vi "move_4.vi"(6 "Array 3":i32[](array[numeric]), 7 "Array 6":i32[](array[numeric]), 9 "Array in":i32[](array[numeric]), 10 "Enum 4":T1(ring), 11 "Enum in":enum16{"move4", "move4_1", "move4_2"}(ring)) -> (1 "Array out":i32[](array[numeric]), 2 "Enum 3":T2(ring), 3 "Enum out":enum16{"move4", "move4_1", "move4_2"}(ring), 4 "Array 4":i32[](array[numeric]), 5 "Array 5":i32[](array[numeric]))   [LabVIEW 2016]
uses:
  <vilib>/NXT/Block Support/NXT_OutputPort.ctl
  <vilib>/NXT/NXTIO Xnodes/NXTIONodeSubVIs/NXTStopMotors.vi
  <vilib>/NXT/NXTIO Xnodes/NXTIONodeSubVIs/NXTMotorRunDistance.vi
  <vilib>/NXT/NXTIO Xnodes/NXTIONodeSubVIs/LEGOMotorStatus.vi
  <vilib>/NXT/NXTIO Xnodes/NXTIONodeSubVIs/NXTMoveMotors.vi
  <vilib>/NXT/NXTIO Xnodes/NXTIONodeSubVIs/LEGOResetMotors.vi
  <vilib>/NXT/Subs/LVHSConnector.ctl
  <vilib>/NXT/NXTIO Xnodes/AddressXNode/NXTIOAddress.xnode
  <vilib>/NXT/NXTIO Xnodes/NXTIOXNode/NXTIO.xnode
  <vilib>/NXT/LegoClasses/BrickReference/BrickReference.lvclass
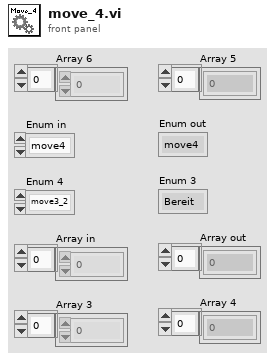
[diagram p1: front panel]
types:
  T1 = enum16{"move3_2", "move3_3", "move3_4", "move3_5"}
  T2 = enum16{"Bereit", "Move 1", "Reference_pos", "Wait", "row1_check", "row2_check", "row3_check", "return", "move2", "move3", "move4", "move5", "end"}
  T3 = enum16{"forward", "right", "mark", "pause", "up", "return", "end"}
  T4 = typedef "NXT_OutputPort.ctl" = u8
  T5 = cluster{"Output Port":T4, "Output Port 2":T4, "Output Port 3":T4}
  T6 = enum16{"forward", "mark", "pause", "up", "return", "end"}
  T7 = typedef "LVHSConnector.ctl" = refnum<class "BrickReference.lvclass">
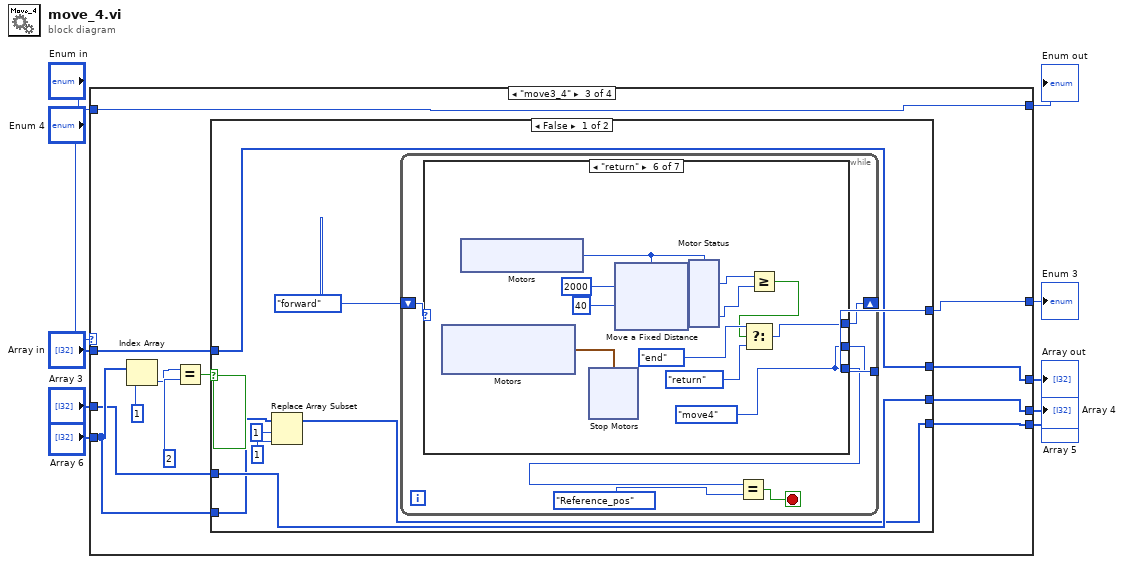
[diagram p0: block diagram]
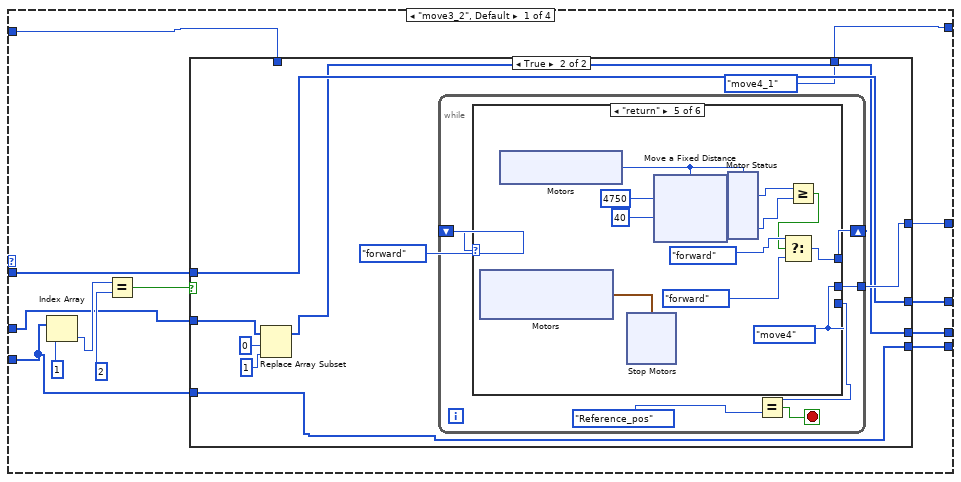
[diagram p2: hidden frame]
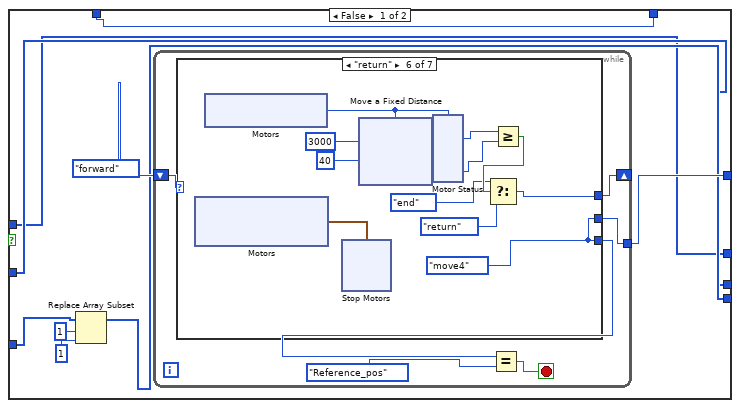
[diagram p3: hidden frame]
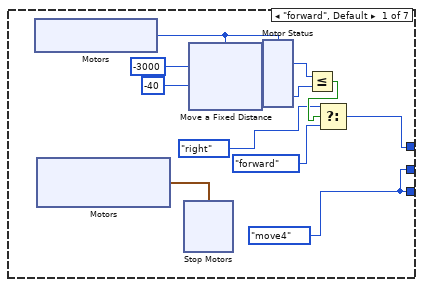
[diagram p4: hidden frame]
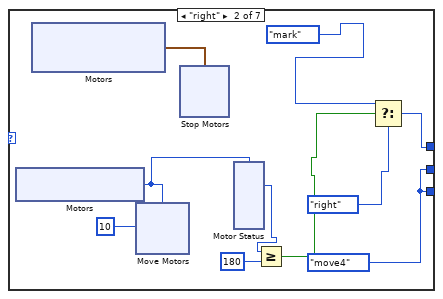
[diagram p5: hidden frame]
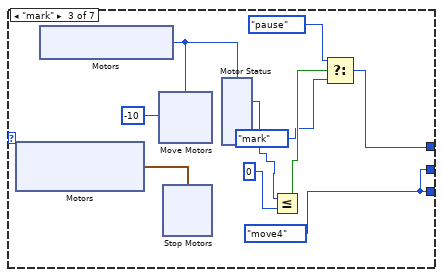
[diagram p6: hidden frame]
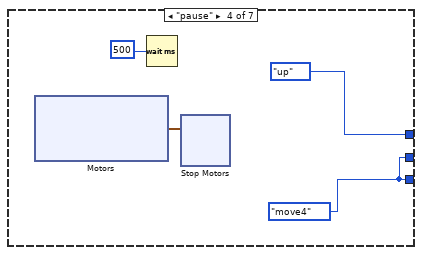
[diagram p7: hidden frame]
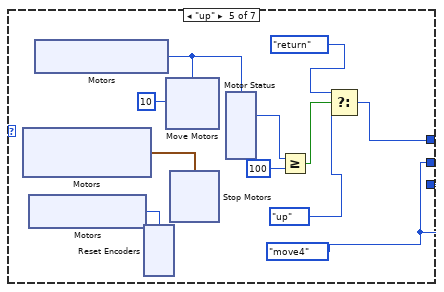
[diagram p8: hidden frame]
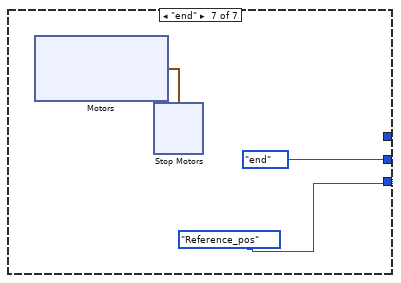
[diagram p9: hidden frame]
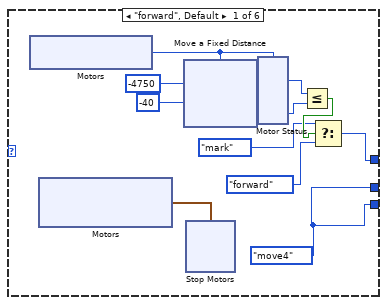
[diagram p10: hidden frame]
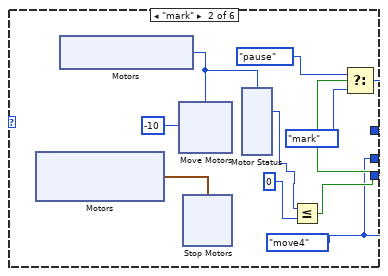
[diagram p11: hidden frame]
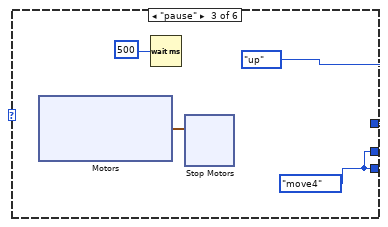
[diagram p12: hidden frame]
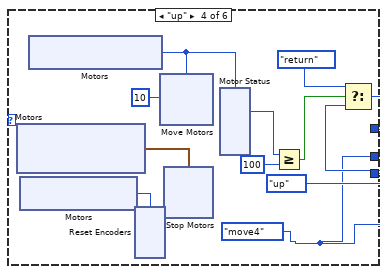
[diagram p13: hidden frame]
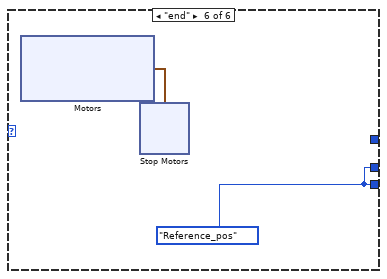
[diagram p14: hidden frame]
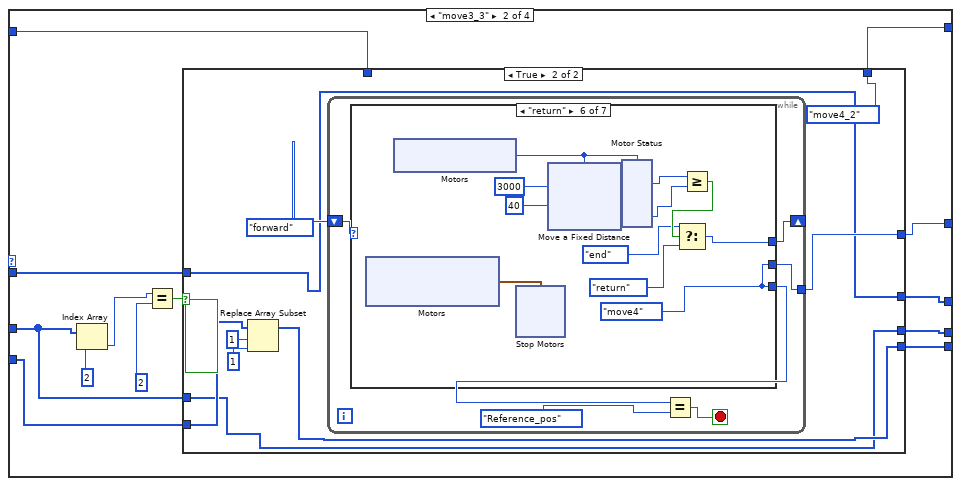
[diagram p15: hidden frame]
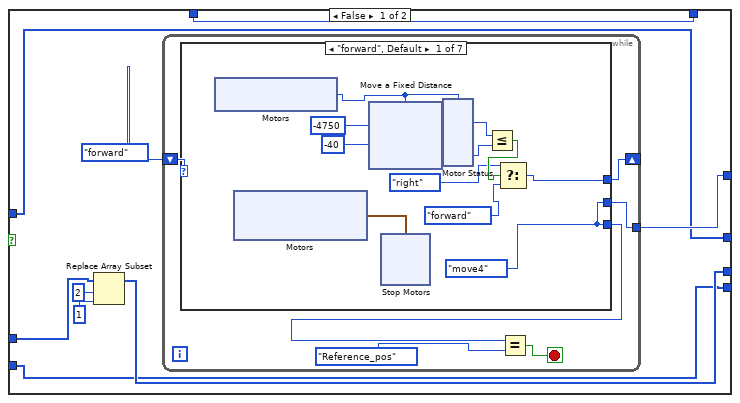
[diagram p16: hidden frame]
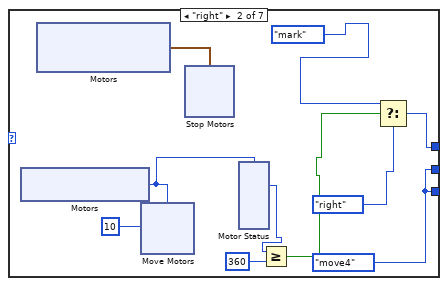
[diagram p17: hidden frame]
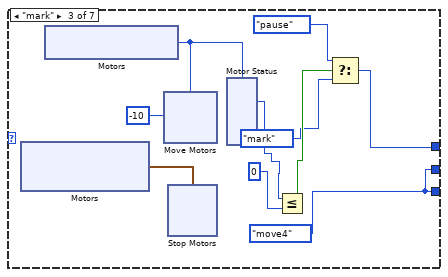
[diagram p18: hidden frame]
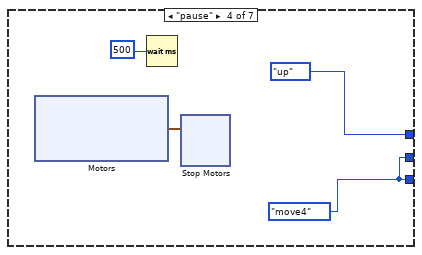
[diagram p19: hidden frame]
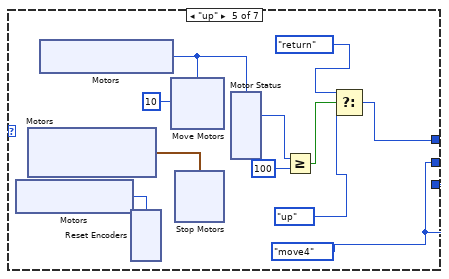
[diagram p20: hidden frame]
diagram:
  n1 = case shown="\"move3_4\"" "Enum 4" {
    tunnel: [w22 w417 w844 w1236] -> w2
    tunnel: [w12 w408 w835 w1227] -> w3
    tunnel: "Enum in" -> [w11 w407 w835 w1227]
    tunnel: "Array 6" -> [w18 w412 w840 w1230]
    tunnel: [w17 w411 w841 w1231] -> w6
    tunnel: [w16 w413 w839 w1228] -> w7
    tunnel: "Array 3" -> [w15 w414 w838 w1229]
    tunnel: [w14 w410 w837 w1233] -> w9
    tunnel: "Array in" -> [w13 w409 w836 w1232]
    frame "move3_2", Default {
      n2 = Index Array(array=w18, index=1) -> (element=w20:i32)
      n3 = Equal?(x=w20, y=2 ("element")) -> (x = y?=w19:bool)
      n4 = case shown="True" w19 {
        tunnel: [w31 w239] -> w22
        tunnel: w18 -> [w29 w233]
        tunnel: [w28 w233] -> w17
        tunnel: [w27 w234] -> w16
        tunnel: w15 -> [w27 w235]
        tunnel: [w26 w236] -> w14
        tunnel: w13 -> [w26 w236]
        tunnel: [w24 enum16{"move4", "move4_1", "move4_2"}."move4_1"] -> w12
        tunnel: w11 -> [w24 _]
        frame False {
          n5 = Replace Array Subset(array=w29, new element=1 ("new element/subarray"), index=1) -> (w28:i32[])
          n6 = while {
            shift-right: [w34] -> _
            shift-left: T3."forward" -> [w35]
            tunnel: [w33] -> w31
            stop <- w37 stop-if-true
            n7 = case shown="\"return\"" w35 {
              tunnel: [w39 w76 w108 T3."up" w151 w187 _] -> w34
              tunnel: [w48 w75 w107 w139 w150 w196 T2."Reference_pos"] -> w38
              tunnel: [w48 w75 w107 w139 w150 w196 T2."end"] -> w33
              frame "forward", Default {
                w43 = -3000 ("Distance 1")
                w48 = T2."move4"
                n8 = xnode "Motors"() -> ("Motor"=w45:T4)
                n9 = xnode "Motors"() -> ("Motor"=w49:cluster{"Port":T4, "Port":T4})
                n10 = xnode "Stop Motors"("Motors"=w49) -> ()  [unwired: 1 in, 1 out]
                n11 = xnode "Move a Fixed Distance"("Speed 1"=i8 -40, "Distance 1"=w43, "Motors"=w45) -> ("NXT/EV3"=w44:T7)  [unwired: 1 in]
                n12 = xnode "Motor Status"("Motors"=w45, "NXT/EV3"=w44) -> ("Position 1"=w46:i32)  [unwired: 2 out]
                n13 = Less Or Equal?(x=w46, y=w43) -> (x <= y?=w42:bool)
                n14 = Select(t=T3."right", s=w42, f=T3."forward") -> (s? t:f=w39:T3)
              }
              frame "right" {
                w75 = T2."move4"
                n15 = xnode "Motors"() -> ("Motor"=w84:T4)
                n16 = xnode "Motors"() -> ("Motor"=w83:cluster{"Port":T4, "Port":T4})
                n17 = xnode "Move Motors"("Power/Speed 1"=i8 10, "Motors"=w84) -> ()  [unwired: 1 in, 1 out]
                n18 = xnode "Stop Motors"("Motors"=w83) -> ()  [unwired: 1 in, 1 out]
                n19 = xnode "Motor Status"("Motors"=w84) -> ("Position 1"=w81:i32)  [unwired: 1 in, 2 out]
                n20 = Greater Or Equal?(x=w81, y=180) -> (x >= y?=w80:bool)
                n21 = Select(t=T3."mark", s=w80, f=T3."right") -> (s? t:f=w76:T3)
              }
              frame "mark" {
                w107 = T2."move4"
                n22 = xnode "Motors"() -> ("Motor"=w116:cluster{"Port":T4, "Port":T4})
                n23 = xnode "Motors"() -> ("Motor"=w114:T4)
                n24 = xnode "Move Motors"("Power/Speed 1"=i8 -10, "Motors"=w114) -> ()  [unwired: 1 in, 1 out]
                n25 = xnode "Stop Motors"("Motors"=w116) -> ()  [unwired: 1 in, 1 out]
                n26 = xnode "Motor Status"("Motors"=w114) -> ("Position 1"=w113:i32)  [unwired: 1 in, 2 out]
                n27 = Less Or Equal?(x=w113, y=0) -> (x <= y?=w111:bool)
                n28 = Select(t=T3."pause", s=w111, f=T3."mark") -> (s? t:f=w108:T3)
              }
              frame "pause" {
                w139 = T2."move4"
                n29 = xnode "Motors"() -> ("Motor"=w142:cluster{"Port":T4, "Port":T4, "Port":T4})
                n30 = Wait (ms)(milliseconds to wait=u32 500 ("millisecond timer value")) -> ()  [unwired: 1 out]
                n31 = xnode "Stop Motors"("Motors"=w142) -> ()  [unwired: 1 in, 1 out]
              }
              frame "up" {
                w150 = T2."move4"
                n32 = xnode "Motors"() -> ("Motor"=w158:cluster{"Port":T4, "Port":T4})
                n33 = xnode "Motors"() -> ("Motor"=w149:T4)
                n34 = xnode "Motors"() -> ("Motor"=w155:T4)
                n35 = xnode "Reset Encoders"("Motors"=w149) -> ()  [unwired: 1 in, 1 out]
                n36 = xnode "Move Motors"("Power/Speed 1"=i8 10, "Motors"=w155) -> ()  [unwired: 1 in, 1 out]
                n37 = xnode "Stop Motors"("Motors"=w158) -> ()  [unwired: 1 in, 1 out]
                n38 = xnode "Motor Status"("Motors"=w155) -> ("Position 1"=w156:i32)  [unwired: 1 in, 2 out]
                n39 = Greater Or Equal?(x=w156, y=100) -> (x >= y?=w157:bool)
                n40 = Select(t=T3."return", s=w157, f=T3."up") -> (s? t:f=w151:T3)
              }
              frame "return" {
                w191 = 3000 ("Distance 1")
                w196 = T2."move4"
                n41 = xnode "Motors"() -> ("Motor"=w197:cluster{"Port":T4, "Port":T4})
                n42 = xnode "Motors"() -> ("Motor"=w194:T4)
                n43 = xnode "Stop Motors"("Motors"=w197) -> ()  [unwired: 1 in, 1 out]
                n44 = xnode "Move a Fixed Distance"("Speed 1"=i8 40, "Distance 1"=w191, "Motors"=w194) -> ("NXT/EV3"=w193:T7)  [unwired: 1 in]
                n45 = xnode "Motor Status"("Motors"=w194, "NXT/EV3"=w193) -> ("Position 1"=w192:i32)  [unwired: 2 out]
                n46 = Greater Or Equal?(x=w192, y=w191) -> (x >= y?=w190:bool)
                n47 = Select(t=T3."end", s=w190, f=T3."return") -> (s? t:f=w187:T3)
              }
              frame "end" {
                n48 = xnode "Motors"() -> ("Motor"=w224:cluster{"Port":T4, "Port":T4, "Port":T4})
                n49 = xnode "Stop Motors"("Motors"=w224) -> ()  [unwired: 1 in, 1 out]
              }
            }
            n50 = Equal?(x=w38, y=T2."Reference_pos") -> (x = y?=w37:bool)
          }
        }
        frame True {
          n51 = Replace Array Subset(array=w235, new element=1 ("new element/subarray"), index=0) -> (w234:i32[])
          n52 = while {
            shift-right: [w246] -> _
            shift-left: T6."forward" -> [w245]
            tunnel: [w241] -> w239
            stop <- w243 stop-if-true
            n53 = case shown="\"return\"" w245 {
              tunnel: [w247 w290 T6."up" w332 w363 _] -> w246
              tunnel: [w256 w283 w315 w326 w372 w399] -> w244
              tunnel: [w256 w283 w315 w326 w372 w399] -> w241
              frame "forward", Default {
                w251 = -4750 ("Distance 1")
                w256 = T2."move4"
                n54 = xnode "Motors"() -> ("Motor"=w253:T4)
                n55 = xnode "Motors"() -> ("Motor"=w257:cluster{"Port":T4, "Port":T4})
                n56 = xnode "Move a Fixed Distance"("Speed 1"=i8 -40, "Distance 1"=w251, "Motors"=w253) -> ("NXT/EV3"=w252:T7)  [unwired: 1 in]
                n57 = xnode "Stop Motors"("Motors"=w257) -> ()  [unwired: 1 in, 1 out]
                n58 = xnode "Motor Status"("Motors"=w253, "NXT/EV3"=w252) -> ("Position 1"=w254:i32)  [unwired: 2 out]
                n59 = Less Or Equal?(x=w254, y=w251) -> (x <= y?=w250:bool)
                n60 = Select(t=T6."mark", s=w250, f=T6."forward") -> (s? t:f=w247:T6)
              }
              frame "mark" {
                w283 = T2."move4"
                n61 = xnode "Motors"() -> ("Motor"=w292:cluster{"Port":T4, "Port":T4})
                n62 = xnode "Motors"() -> ("Motor"=w287:T4)
                n63 = xnode "Move Motors"("Power/Speed 1"=i8 -10, "Motors"=w287) -> ()  [unwired: 1 in, 1 out]
                n64 = xnode "Stop Motors"("Motors"=w292) -> ()  [unwired: 1 in, 1 out]
                n65 = xnode "Motor Status"("Motors"=w287) -> ("Position 1"=w286:i32)  [unwired: 1 in, 2 out]
                n66 = Less Or Equal?(x=w286, y=0) -> (x <= y?=w284:bool)
                n67 = Select(t=T6."pause", s=w284, f=T6."mark") -> (s? t:f=w290:T6)
              }
              frame "pause" {
                w315 = T2."move4"
                n68 = xnode "Motors"() -> ("Motor"=w318:cluster{"Port":T4, "Port":T4, "Port":T4})
                n69 = Wait (ms)(milliseconds to wait=u32 500 ("millisecond timer value")) -> ()  [unwired: 1 out]
                n70 = xnode "Stop Motors"("Motors"=w318) -> ()  [unwired: 1 in, 1 out]
              }
              frame "up" {
                w326 = T2."move4"
                n71 = xnode "Motors"() -> ("Motor"=w334:cluster{"Port":T4, "Port":T4})
                n72 = xnode "Motors"() -> ("Motor"=w325:T4)
                n73 = xnode "Motors"() -> ("Motor"=w328:T4)
                n74 = xnode "Reset Encoders"("Motors"=w325) -> ()  [unwired: 1 in, 1 out]
                n75 = xnode "Move Motors"("Power/Speed 1"=i8 10, "Motors"=w328) -> ()  [unwired: 1 in, 1 out]
                n76 = xnode "Stop Motors"("Motors"=w334) -> ()  [unwired: 1 in, 1 out]
                n77 = xnode "Motor Status"("Motors"=w328) -> ("Position 1"=w329:i32)  [unwired: 1 in, 2 out]
                n78 = Greater Or Equal?(x=w329, y=100) -> (x >= y?=w333:bool)
                n79 = Select(t=T6."return", s=w333, f=T6."up") -> (s? t:f=w332:T6)
              }
              frame "return" {
                w367 = 4750 ("Distance 1")
                w372 = T2."move4"
                n80 = xnode "Motors"() -> ("Motor"=w373:cluster{"Port":T4, "Port":T4})
                n81 = xnode "Motors"() -> ("Motor"=w370:T4)
                n82 = xnode "Stop Motors"("Motors"=w373) -> ()  [unwired: 1 in, 1 out]
                n83 = xnode "Move a Fixed Distance"("Speed 1"=i8 40, "Distance 1"=w367, "Motors"=w370) -> ("NXT/EV3"=w369:T7)  [unwired: 1 in]
                n84 = xnode "Motor Status"("Motors"=w370, "NXT/EV3"=w369) -> ("Position 1"=w368:i32)  [unwired: 2 out]
                n85 = Greater Or Equal?(x=w368, y=w367) -> (x >= y?=w364:bool)
                n86 = Select(t=T6."forward", s=w364, f=T6."forward") -> (s? t:f=w363:T6)
              }
              frame "end" {
                w399 = T2."Reference_pos"
                n87 = xnode "Motors"() -> ("Motor"=w400:cluster{"Port":T4, "Port":T4, "Port":T4})
                n88 = xnode "Stop Motors"("Motors"=w400) -> ()  [unwired: 1 in, 1 out]
              }
            }
            n89 = Equal?(x=w244, y=T2."Reference_pos") -> (x = y?=w243:bool)
          }
        }
      }
    }
    frame "move3_3" {
      n90 = Index Array(array=w414, index=2) -> (element=w415:i32)
      n91 = Equal?(x=w415, y=2 ("element")) -> (x = y?=w418:bool)
      n92 = case shown="True" w418 {
        tunnel: [w427 w635] -> w417
        tunnel: w414 -> [w424 w630]
        tunnel: [w423 w630] -> w413
        tunnel: w412 -> [w421 w632]
        tunnel: [w421 w631] -> w411
        tunnel: [w422 w629] -> w410
        tunnel: w409 -> [w422 w629]
        tunnel: [w420 enum16{"move4", "move4_1", "move4_2"}."move4_2"] -> w408
        tunnel: w407 -> [w420 _]
        frame False {
          n93 = Replace Array Subset(array=w424, new element=1 ("new element/subarray"), index=2) -> (w423:i32[])
          n94 = while {
            shift-right: [w430] -> _
            shift-left: T3."forward" -> [w431]
            tunnel: [w429] -> w427
            stop <- w433 stop-if-true
            n95 = case shown="\"forward\", Default" w431 {
              tunnel: [w435 w472 w504 T3."up" w547 w583 _] -> w430
              tunnel: [w444 w471 w503 w535 w546 w592 T2."Reference_pos"] -> w434
              tunnel: [w444 w471 w503 w535 w546 w592 T2."end"] -> w429
              frame "forward", Default {
                w440 = -4750 ("Distance 1")
                w444 = T2."move4"
                n96 = xnode "Motors"() -> ("Motor"=w436:T4)
                n97 = xnode "Motors"() -> ("Motor"=w445:cluster{"Port":T4, "Port":T4})
                n98 = xnode "Move a Fixed Distance"("Speed 1"=i8 -40, "Distance 1"=w440, "Motors"=w436) -> ("NXT/EV3"=w441:T7)  [unwired: 1 in]
                n99 = xnode "Stop Motors"("Motors"=w445) -> ()  [unwired: 1 in, 1 out]
                n100 = xnode "Motor Status"("Motors"=w436, "NXT/EV3"=w441) -> ("Position 1"=w442:i32)  [unwired: 2 out]
                n101 = Less Or Equal?(x=w442, y=w440) -> (x <= y?=w439:bool)
                n102 = Select(t=T3."right", s=w439, f=T3."forward") -> (s? t:f=w435:T3)
              }
              frame "right" {
                w471 = T2."move4"
                n103 = xnode "Motors"() -> ("Motor"=w480:T4)
                n104 = xnode "Motors"() -> ("Motor"=w479:cluster{"Port":T4, "Port":T4})
                n105 = xnode "Move Motors"("Power/Speed 1"=i8 10, "Motors"=w480) -> ()  [unwired: 1 in, 1 out]
                n106 = xnode "Stop Motors"("Motors"=w479) -> ()  [unwired: 1 in, 1 out]
                n107 = xnode "Motor Status"("Motors"=w480) -> ("Position 1"=w477:i32)  [unwired: 1 in, 2 out]
                n108 = Greater Or Equal?(x=w477, y=360) -> (x >= y?=w476:bool)
                n109 = Select(t=T3."mark", s=w476, f=T3."right") -> (s? t:f=w472:T3)
              }
              frame "mark" {
                w503 = T2."move4"
                n110 = xnode "Motors"() -> ("Motor"=w512:cluster{"Port":T4, "Port":T4})
                n111 = xnode "Motors"() -> ("Motor"=w510:T4)
                n112 = xnode "Move Motors"("Power/Speed 1"=i8 -10, "Motors"=w510) -> ()  [unwired: 1 in, 1 out]
                n113 = xnode "Stop Motors"("Motors"=w512) -> ()  [unwired: 1 in, 1 out]
                n114 = xnode "Motor Status"("Motors"=w510) -> ("Position 1"=w509:i32)  [unwired: 1 in, 2 out]
                n115 = Less Or Equal?(x=w509, y=0) -> (x <= y?=w507:bool)
                n116 = Select(t=T3."pause", s=w507, f=T3."mark") -> (s? t:f=w504:T3)
              }
              frame "pause" {
                w535 = T2."move4"
                n117 = xnode "Motors"() -> ("Motor"=w538:cluster{"Port":T4, "Port":T4, "Port":T4})
                n118 = Wait (ms)(milliseconds to wait=u32 500 ("millisecond timer value")) -> ()  [unwired: 1 out]
                n119 = xnode "Stop Motors"("Motors"=w538) -> ()  [unwired: 1 in, 1 out]
              }
              frame "up" {
                w546 = T2."move4"
                n120 = xnode "Motors"() -> ("Motor"=w545:T4)
                n121 = xnode "Motors"() -> ("Motor"=w554:cluster{"Port":T4, "Port":T4})
                n122 = xnode "Motors"() -> ("Motor"=w551:T4)
                n123 = xnode "Reset Encoders"("Motors"=w545) -> ()  [unwired: 1 in, 1 out]
                n124 = xnode "Move Motors"("Power/Speed 1"=i8 10, "Motors"=w551) -> ()  [unwired: 1 in, 1 out]
                n125 = xnode "Stop Motors"("Motors"=w554) -> ()  [unwired: 1 in, 1 out]
                n126 = xnode "Motor Status"("Motors"=w551) -> ("Position 1"=w552:i32)  [unwired: 1 in, 2 out]
                n127 = Greater Or Equal?(x=w552, y=100) -> (x >= y?=w553:bool)
                n128 = Select(t=T3."return", s=w553, f=T3."up") -> (s? t:f=w547:T3)
              }
              frame "return" {
                w587 = 4000 ("Distance 1")
                w592 = T2."move4"
                n129 = xnode "Motors"() -> ("Motor"=w593:cluster{"Port":T4, "Port":T4})
                n130 = xnode "Motors"() -> ("Motor"=w590:T4)
                n131 = xnode "Stop Motors"("Motors"=w593) -> ()  [unwired: 1 in, 1 out]
                n132 = xnode "Move a Fixed Distance"("Speed 1"=i8 40, "Distance 1"=w587, "Motors"=w590) -> ("NXT/EV3"=w589:T7)  [unwired: 1 in]
                n133 = xnode "Motor Status"("Motors"=w590, "NXT/EV3"=w589) -> ("Position 1"=w588:i32)  [unwired: 2 out]
                n134 = Greater Or Equal?(x=w588, y=w587) -> (x >= y?=w586:bool)
                n135 = Select(t=T3."end", s=w586, f=T3."return") -> (s? t:f=w583:T3)
              }
              frame "end" {
                n136 = xnode "Motors"() -> ("Motor"=w620:cluster{"Port":T4, "Port":T4, "Port":T4})
                n137 = xnode "Stop Motors"("Motors"=w620) -> ()  [unwired: 1 in, 1 out]
              }
            }
            n138 = Equal?(x=w434, y=T2."Reference_pos") -> (x = y?=w433:bool)
          }
        }
        frame True {
          n139 = Replace Array Subset(array=w632, new element=1 ("new element/subarray"), index=1) -> (w631:i32[])
          n140 = while {
            shift-right: [w638] -> _
            shift-left: T3."forward" -> [w639]
            tunnel: [w637] -> w635
            stop <- w641 stop-if-true
            n141 = case shown="\"return\"" w639 {
              tunnel: [w643 w680 w712 T3."up" w755 w791 _] -> w638
              tunnel: [w652 w679 w711 w743 w754 w800 w827] -> w642
              tunnel: [w652 w679 w711 w743 w754 w800 w827] -> w637
              frame "forward", Default {
                w648 = -3000 ("Distance 1")
                w652 = T2."move4"
                n142 = xnode "Motors"() -> ("Motor"=w653:cluster{"Port":T4, "Port":T4})
                n143 = xnode "Motors"() -> ("Motor"=w647:T4)
                n144 = xnode "Stop Motors"("Motors"=w653) -> ()  [unwired: 1 in, 1 out]
                n145 = xnode "Move a Fixed Distance"("Speed 1"=i8 -40, "Distance 1"=w648, "Motors"=w647) -> ("NXT/EV3"=w649:T7)  [unwired: 1 in]
                n146 = xnode "Motor Status"("Motors"=w647, "NXT/EV3"=w649) -> ("Position 1"=w650:i32)  [unwired: 2 out]
                n147 = Less Or Equal?(x=w650, y=w648) -> (x <= y?=w644:bool)
                n148 = Select(t=T3."right", s=w644, f=T3."forward") -> (s? t:f=w643:T3)
              }
              frame "right" {
                w679 = T2."move4"
                n149 = xnode "Motors"() -> ("Motor"=w688:T4)
                n150 = xnode "Motors"() -> ("Motor"=w687:cluster{"Port":T4, "Port":T4})
                n151 = xnode "Move Motors"("Power/Speed 1"=i8 10, "Motors"=w688) -> ()  [unwired: 1 in, 1 out]
                n152 = xnode "Stop Motors"("Motors"=w687) -> ()  [unwired: 1 in, 1 out]
                n153 = xnode "Motor Status"("Motors"=w688) -> ("Position 1"=w685:i32)  [unwired: 1 in, 2 out]
                n154 = Greater Or Equal?(x=w685, y=180) -> (x >= y?=w684:bool)
                n155 = Select(t=T3."mark", s=w684, f=T3."right") -> (s? t:f=w680:T3)
              }
              frame "mark" {
                w711 = T2."move4"
                n156 = xnode "Motors"() -> ("Motor"=w720:cluster{"Port":T4, "Port":T4})
                n157 = xnode "Motors"() -> ("Motor"=w718:T4)
                n158 = xnode "Move Motors"("Power/Speed 1"=i8 -10, "Motors"=w718) -> ()  [unwired: 1 in, 1 out]
                n159 = xnode "Stop Motors"("Motors"=w720) -> ()  [unwired: 1 in, 1 out]
                n160 = xnode "Motor Status"("Motors"=w718) -> ("Position 1"=w717:i32)  [unwired: 1 in, 2 out]
                n161 = Less Or Equal?(x=w717, y=0) -> (x <= y?=w715:bool)
                n162 = Select(t=T3."pause", s=w715, f=T3."mark") -> (s? t:f=w712:T3)
              }
              frame "pause" {
                w743 = T2."move4"
                n163 = xnode "Motors"() -> ("Motor"=w746:cluster{"Port":T4, "Port":T4, "Port":T4})
                n164 = Wait (ms)(milliseconds to wait=u32 500 ("millisecond timer value")) -> ()  [unwired: 1 out]
                n165 = xnode "Stop Motors"("Motors"=w746) -> ()  [unwired: 1 in, 1 out]
              }
              frame "up" {
                w754 = T2."move4"
                n166 = xnode "Motors"() -> ("Motor"=w753:T4)
                n167 = xnode "Motors"() -> ("Motor"=w762:cluster{"Port":T4, "Port":T4})
                n168 = xnode "Motors"() -> ("Motor"=w759:T4)
                n169 = xnode "Reset Encoders"("Motors"=w753) -> ()  [unwired: 1 in, 1 out]
                n170 = xnode "Move Motors"("Power/Speed 1"=i8 10, "Motors"=w759) -> ()  [unwired: 1 in, 1 out]
                n171 = xnode "Stop Motors"("Motors"=w762) -> ()  [unwired: 1 in, 1 out]
                n172 = xnode "Motor Status"("Motors"=w759) -> ("Position 1"=w760:i32)  [unwired: 1 in, 2 out]
                n173 = Greater Or Equal?(x=w760, y=100) -> (x >= y?=w761:bool)
                n174 = Select(t=T3."return", s=w761, f=T3."up") -> (s? t:f=w755:T3)
              }
              frame "return" {
                w795 = 3000 ("Distance 1")
                w800 = T2."move4"
                n175 = xnode "Motors"() -> ("Motor"=w801:cluster{"Port":T4, "Port":T4})
                n176 = xnode "Motors"() -> ("Motor"=w798:T4)
                n177 = xnode "Stop Motors"("Motors"=w801) -> ()  [unwired: 1 in, 1 out]
                n178 = xnode "Move a Fixed Distance"("Speed 1"=i8 40, "Distance 1"=w795, "Motors"=w798) -> ("NXT/EV3"=w797:T7)  [unwired: 1 in]
                n179 = xnode "Motor Status"("Motors"=w798, "NXT/EV3"=w797) -> ("Position 1"=w796:i32)  [unwired: 2 out]
                n180 = Greater Or Equal?(x=w796, y=w795) -> (x >= y?=w794:bool)
                n181 = Select(t=T3."end", s=w794, f=T3."return") -> (s? t:f=w791:T3)
              }
              frame "end" {
                w827 = T2."Reference_pos"
                n182 = xnode "Motors"() -> ("Motor"=w828:cluster{"Port":T4, "Port":T4, "Port":T4})
                n183 = xnode "Stop Motors"("Motors"=w828) -> ()  [unwired: 1 in, 1 out]
              }
            }
            n184 = Equal?(x=w642, y=T2."Reference_pos") -> (x = y?=w641:bool)
          }
        }
      }
    }
    frame "move3_4" {
      n185 = Index Array(array=w840, index=1) -> (element=w842:i32)
      n186 = Equal?(x=w842, y=2 ("element")) -> (x = y?=w845:bool)
      n187 = case shown="False" w845 {
        tunnel: [w853 w1059] -> w844
        tunnel: [w847 w1053] -> w841
        tunnel: w840 -> [w848 w1053]
        tunnel: [w852 w1054] -> w839
        tunnel: w838 -> [w852 w1054]
        tunnel: [w851 w1055] -> w837
        tunnel: w836 -> [w851 w1058]
        frame False {
          n188 = Replace Array Subset(array=w848, new element=1 ("new element/subarray"), index=1) -> (w847:i32[])
          n189 = while {
            shift-right: [w856] -> _
            shift-left: T3."forward" -> [w857]
            tunnel: [w855] -> w853
            stop <- w859 stop-if-true
            n190 = case shown="\"return\"" w857 {
              tunnel: [w861 w898 w930 w961 w972 w1008 _] -> w856
              tunnel: [w870 w897 w929 w963 w971 w1017 T2."Reference_pos"] -> w860
              tunnel: [w870 w897 w929 w963 w971 w1017 T2."end"] -> w855
              frame "forward", Default {
                w866 = -3000 ("Distance 1")
                w870 = T2."move4"
                n191 = xnode "Motors"() -> ("Motor"=w871:cluster{"Port":T4, "Port":T4})
                n192 = xnode "Motors"() -> ("Motor"=w865:T4)
                n193 = xnode "Stop Motors"("Motors"=w871) -> ()  [unwired: 1 in, 1 out]
                n194 = xnode "Move a Fixed Distance"("Speed 1"=i8 -40, "Distance 1"=w866, "Motors"=w865) -> ("NXT/EV3"=w867:T7)  [unwired: 1 in]
                n195 = xnode "Motor Status"("Motors"=w865, "NXT/EV3"=w867) -> ("Position 1"=w868:i32)  [unwired: 2 out]
                n196 = Less Or Equal?(x=w868, y=w866) -> (x <= y?=w864:bool)
                n197 = Select(t=T3."right", s=w864, f=T3."forward") -> (s? t:f=w861:T3)
              }
              frame "right" {
                w897 = T2."move4"
                n198 = xnode "Motors"() -> ("Motor"=w906:T4)
                n199 = xnode "Motors"() -> ("Motor"=w905:cluster{"Port":T4, "Port":T4})
                n200 = xnode "Move Motors"("Power/Speed 1"=i8 10, "Motors"=w906) -> ()  [unwired: 1 in, 1 out]
                n201 = xnode "Stop Motors"("Motors"=w905) -> ()  [unwired: 1 in, 1 out]
                n202 = xnode "Motor Status"("Motors"=w906) -> ("Position 1"=w903:i32)  [unwired: 1 in, 2 out]
                n203 = Greater Or Equal?(x=w903, y=220) -> (x >= y?=w902:bool)
                n204 = Select(t=T3."mark", s=w902, f=T3."right") -> (s? t:f=w898:T3)
              }
              frame "mark" {
                w929 = T2."move4"
                n205 = xnode "Motors"() -> ("Motor"=w938:cluster{"Port":T4, "Port":T4})
                n206 = xnode "Motors"() -> ("Motor"=w936:T4)
                n207 = xnode "Move Motors"("Power/Speed 1"=i8 -10, "Motors"=w936) -> ()  [unwired: 1 in, 1 out]
                n208 = xnode "Stop Motors"("Motors"=w938) -> ()  [unwired: 1 in, 1 out]
                n209 = xnode "Motor Status"("Motors"=w936) -> ("Position 1"=w935:i32)  [unwired: 1 in, 2 out]
                n210 = Less Or Equal?(x=w935, y=0) -> (x <= y?=w933:bool)
                n211 = Select(t=T3."pause", s=w933, f=T3."mark") -> (s? t:f=w930:T3)
              }
              frame "pause" {
                w963 = T2."move4"
                n212 = xnode "Motors"() -> ("Motor"=w962:cluster{"Port":T4, "Port":T4})
                n213 = call "x1_move4.vi"() -> ("Enum"=w961:T3)  [unwired: 1 in]
                n214 = xnode "Stop Motors"("Motors"=w962) -> ()  [unwired: 1 in, 1 out]
              }
              frame "up" {
                w971 = T2."move4"
                n215 = xnode "Motors"() -> ("Motor"=w970:T4)
                n216 = xnode "Motors"() -> ("Motor"=w979:cluster{"Port":T4, "Port":T4})
                n217 = xnode "Motors"() -> ("Motor"=w976:T4)
                n218 = xnode "Reset Encoders"("Motors"=w970) -> ()  [unwired: 1 in, 1 out]
                n219 = xnode "Move Motors"("Power/Speed 1"=i8 10, "Motors"=w976) -> ()  [unwired: 1 in, 1 out]
                n220 = xnode "Stop Motors"("Motors"=w979) -> ()  [unwired: 1 in, 1 out]
                n221 = xnode "Motor Status"("Motors"=w976) -> ("Position 1"=w977:i32)  [unwired: 1 in, 2 out]
                n222 = Greater Or Equal?(x=w977, y=100) -> (x >= y?=w978:bool)
                n223 = Select(t=T3."return", s=w978, f=T3."up") -> (s? t:f=w972:T3)
              }
              frame "return" {
                w1012 = 2000 ("Distance 1")
                w1017 = T2."move4"
                n224 = xnode "Motors"() -> ("Motor"=w1018:cluster{"Port":T4, "Port":T4})
                n225 = xnode "Motors"() -> ("Motor"=w1015:T4)
                n226 = xnode "Stop Motors"("Motors"=w1018) -> ()  [unwired: 1 in, 1 out]
                n227 = xnode "Move a Fixed Distance"("Speed 1"=i8 40, "Distance 1"=w1012, "Motors"=w1015) -> ("NXT/EV3"=w1014:T7)  [unwired: 1 in]
                n228 = xnode "Motor Status"("Motors"=w1015, "NXT/EV3"=w1014) -> ("Position 1"=w1013:i32)  [unwired: 2 out]
                n229 = Greater Or Equal?(x=w1013, y=w1012) -> (x >= y?=w1009:bool)
                n230 = Select(t=T3."end", s=w1009, f=T3."return") -> (s? t:f=w1008:T3)
              }
              frame "end" {
                n231 = xnode "Motors"() -> ("Motor"=w1045:cluster{"Port":T4, "Port":T4, "Port":T4})
                n232 = xnode "Stop Motors"("Motors"=w1045) -> ()  [unwired: 1 in, 1 out]
              }
            }
            n233 = Equal?(x=w860, y=T2."Reference_pos") -> (x = y?=w859:bool)
          }
        }
        frame True {
          n234 = Replace Array Subset(array=w1058, new element=2 ("new element/subarray"), index=1) -> (w1055:i32[])
          n235 = while {
            shift-right: [w1066] -> _
            shift-left: T6."forward" -> [w1065]
            tunnel: [w1061] -> w1059
            stop <- w1063 stop-if-true
            n236 = case shown="\"pause\"" w1065 {
              tunnel: [w1067 w1110 T6."up" w1152 w1184 _] -> w1066
              tunnel: [w1076 w1103 w1135 w1146 w1192 w1219] -> w1064
              tunnel: [w1076 w1103 w1135 w1146 w1192 w1219] -> w1061
              frame "forward", Default {
                w1072 = -6500 ("Distance 1")
                w1076 = T2."move4"
                n237 = xnode "Motors"() -> ("Motor"=w1071:T4)
                n238 = xnode "Motors"() -> ("Motor"=w1077:cluster{"Port":T4, "Port":T4})
                n239 = xnode "Stop Motors"("Motors"=w1077) -> ()  [unwired: 1 in, 1 out]
                n240 = xnode "Move a Fixed Distance"("Speed 1"=i8 -40, "Distance 1"=w1072, "Motors"=w1071) -> ("NXT/EV3"=w1073:T7)  [unwired: 1 in]
                n241 = xnode "Motor Status"("Motors"=w1071, "NXT/EV3"=w1073) -> ("Position 1"=w1074:i32)  [unwired: 2 out]
                n242 = Less Or Equal?(x=w1074, y=w1072) -> (x <= y?=w1070:bool)
                n243 = Select(t=T6."mark", s=w1070, f=T6."forward") -> (s? t:f=w1067:T6)
              }
              frame "mark" {
                w1103 = T2."move4"
                n244 = xnode "Motors"() -> ("Motor"=w1112:cluster{"Port":T4, "Port":T4})
                n245 = xnode "Motors"() -> ("Motor"=w1107:T4)
                n246 = xnode "Move Motors"("Power/Speed 1"=i8 -10, "Motors"=w1107) -> ()  [unwired: 1 in, 1 out]
                n247 = xnode "Stop Motors"("Motors"=w1112) -> ()  [unwired: 1 in, 1 out]
                n248 = xnode "Motor Status"("Motors"=w1107) -> ("Position 1"=w1106:i32)  [unwired: 1 in, 2 out]
                n249 = Less Or Equal?(x=w1106, y=0) -> (x <= y?=w1104:bool)
                n250 = Select(t=T6."pause", s=w1104, f=T6."mark") -> (s? t:f=w1110:T6)
              }
              frame "pause" {
                w1135 = T2."move4"
                n251 = xnode "Motors"() -> ("Motor"=w1138:cluster{"Port":T4, "Port":T4, "Port":T4})
                n252 = Wait (ms)(milliseconds to wait=u32 500 ("millisecond timer value")) -> ()  [unwired: 1 out]
                n253 = xnode "Stop Motors"("Motors"=w1138) -> ()  [unwired: 1 in, 1 out]
              }
              frame "up" {
                w1146 = T2."move4"
                n254 = xnode "Motors"() -> ("Motor"=w1154:cluster{"Port":T4, "Port":T4})
                n255 = xnode "Motors"() -> ("Motor"=w1145:T4)
                n256 = xnode "Motors"() -> ("Motor"=w1148:T4)
                n257 = xnode "Reset Encoders"("Motors"=w1145) -> ()  [unwired: 1 in, 1 out]
                n258 = xnode "Move Motors"("Power/Speed 1"=i8 10, "Motors"=w1148) -> ()  [unwired: 1 in, 1 out]
                n259 = xnode "Stop Motors"("Motors"=w1154) -> ()  [unwired: 1 in, 1 out]
                n260 = xnode "Motor Status"("Motors"=w1148) -> ("Position 1"=w1149:i32)  [unwired: 1 in, 2 out]
                n261 = Greater Or Equal?(x=w1149, y=100) -> (x >= y?=w1153:bool)
                n262 = Select(t=T6."return", s=w1153, f=T6."up") -> (s? t:f=w1152:T6)
              }
              frame "return" {
                w1187 = 6500 ("Distance 1")
                w1192 = T2."move4"
                n263 = xnode "Motors"() -> ("Motor"=w1193:cluster{"Port":T4, "Port":T4})
                n264 = xnode "Motors"() -> ("Motor"=w1190:T4)
                n265 = xnode "Stop Motors"("Motors"=w1193) -> ()  [unwired: 1 in, 1 out]
                n266 = xnode "Move a Fixed Distance"("Speed 1"=i8 40, "Distance 1"=w1187, "Motors"=w1190) -> ("NXT/EV3"=w1189:T7)  [unwired: 1 in]
                n267 = xnode "Motor Status"("Motors"=w1190, "NXT/EV3"=w1189) -> ("Position 1"=w1188:i32)  [unwired: 2 out]
                n268 = Greater Or Equal?(x=w1188, y=w1187) -> (x >= y?=w1183:bool)
                n269 = Select(t=T6."end", s=w1183, f=T6."return") -> (s? t:f=w1184:T6)
              }
              frame "end" {
                w1219 = T2."Reference_pos"
                n270 = xnode "Motors"() -> ("Motor"=w1220:cluster{"Port":T4, "Port":T4, "Port":T4})
                n271 = xnode "Stop Motors"("Motors"=w1220) -> ()  [unwired: 1 in, 1 out]
              }
            }
            n272 = Equal?(x=w1064, y=T2."Reference_pos") -> (x = y?=w1063:bool)
          }
        }
      }
    }
    frame "move3_5" {
      n273 = Index Array(array=w1229, index=2) -> (element=w1234:i32)
      n274 = Equal?(x=w1234, y=2 ("element")) -> (x = y?=w1237:bool)
      n275 = case shown="True" w1237 {
        tunnel: [w1245 w1452] -> w1236
        tunnel: [w1244 w1446] -> w1233
        tunnel: w1232 -> [w1244 w1446]
        tunnel: [w1243 w1448] -> w1231
        tunnel: w1230 -> [w1243 w1449]
        tunnel: w1229 -> [w1240 w1447]
        tunnel: [w1239 w1447] -> w1228
        frame False {
          n276 = Replace Array Subset(array=w1240, new element=1 ("new element/subarray"), index=2) -> (w1239:i32[])
          n277 = while {
            shift-right: [w1248] -> _
            shift-left: T3."forward" -> [w1249]
            tunnel: [w1247] -> w1245
            stop <- w1251 stop-if-true
            n278 = case shown="\"return\"" w1249 {
              tunnel: [w1253 w1290 w1322 T3."up" w1365 w1401 _] -> w1248
              tunnel: [w1262 w1289 w1321 w1353 w1364 w1410 T2."Reference_pos"] -> w1252
              tunnel: [w1262 w1289 w1321 w1353 w1364 w1410 T2."end"] -> w1247
              frame "forward", Default {
                w1258 = -4750 ("Distance 1")
                w1262 = T2."move4"
                n279 = xnode "Motors"() -> ("Motor"=w1263:cluster{"Port":T4, "Port":T4})
                n280 = xnode "Motors"() -> ("Motor"=w1257:T4)
                n281 = xnode "Stop Motors"("Motors"=w1263) -> ()  [unwired: 1 in, 1 out]
                n282 = xnode "Move a Fixed Distance"("Speed 1"=i8 -40, "Distance 1"=w1258, "Motors"=w1257) -> ("NXT/EV3"=w1259:T7)  [unwired: 1 in]
                n283 = xnode "Motor Status"("Motors"=w1257, "NXT/EV3"=w1259) -> ("Position 1"=w1260:i32)  [unwired: 2 out]
                n284 = Less Or Equal?(x=w1260, y=w1258) -> (x <= y?=w1256:bool)
                n285 = Select(t=T3."right", s=w1256, f=T3."forward") -> (s? t:f=w1253:T3)
              }
              frame "right" {
                w1289 = T2."move4"
                n286 = xnode "Motors"() -> ("Motor"=w1298:T4)
                n287 = xnode "Motors"() -> ("Motor"=w1297:cluster{"Port":T4, "Port":T4})
                n288 = xnode "Move Motors"("Power/Speed 1"=i8 10, "Motors"=w1298) -> ()  [unwired: 1 in, 1 out]
                n289 = xnode "Stop Motors"("Motors"=w1297) -> ()  [unwired: 1 in, 1 out]
                n290 = xnode "Motor Status"("Motors"=w1298) -> ("Position 1"=w1295:i32)  [unwired: 1 in, 2 out]
                n291 = Greater Or Equal?(x=w1295, y=360) -> (x >= y?=w1294:bool)
                n292 = Select(t=T3."mark", s=w1294, f=T3."right") -> (s? t:f=w1290:T3)
              }
              frame "mark" {
                w1321 = T2."move4"
                n293 = xnode "Motors"() -> ("Motor"=w1330:cluster{"Port":T4, "Port":T4})
                n294 = xnode "Motors"() -> ("Motor"=w1328:T4)
                n295 = xnode "Move Motors"("Power/Speed 1"=i8 -10, "Motors"=w1328) -> ()  [unwired: 1 in, 1 out]
                n296 = xnode "Stop Motors"("Motors"=w1330) -> ()  [unwired: 1 in, 1 out]
                n297 = xnode "Motor Status"("Motors"=w1328) -> ("Position 1"=w1327:i32)  [unwired: 1 in, 2 out]
                n298 = Less Or Equal?(x=w1327, y=0) -> (x <= y?=w1325:bool)
                n299 = Select(t=T3."pause", s=w1325, f=T3."mark") -> (s? t:f=w1322:T3)
              }
              frame "pause" {
                w1353 = T2."move4"
                n300 = xnode "Motors"() -> ("Motor"=w1356:cluster{"Port":T4, "Port":T4, "Port":T4})
                n301 = Wait (ms)(milliseconds to wait=u32 500 ("millisecond timer value")) -> ()  [unwired: 1 out]
                n302 = xnode "Stop Motors"("Motors"=w1356) -> ()  [unwired: 1 in, 1 out]
              }
              frame "up" {
                w1364 = T2."move4"
                n303 = xnode "Motors"() -> ("Motor"=w1369:T4)
                n304 = xnode "Motors"() -> ("Motor"=w1372:cluster{"Port":T4, "Port":T4})
                n305 = xnode "Motors"() -> ("Motor"=w1363:T4)
                n306 = xnode "Reset Encoders"("Motors"=w1363) -> ()  [unwired: 1 in, 1 out]
                n307 = xnode "Move Motors"("Power/Speed 1"=i8 10, "Motors"=w1369) -> ()  [unwired: 1 in, 1 out]
                n308 = xnode "Stop Motors"("Motors"=w1372) -> ()  [unwired: 1 in, 1 out]
                n309 = xnode "Motor Status"("Motors"=w1369) -> ("Position 1"=w1370:i32)  [unwired: 1 in, 2 out]
                n310 = Greater Or Equal?(x=w1370, y=100) -> (x >= y?=w1371:bool)
                n311 = Select(t=T3."return", s=w1371, f=T3."up") -> (s? t:f=w1365:T3)
              }
              frame "return" {
                w1405 = 4750 ("Distance 1")
                w1410 = T2."move4"
                n312 = xnode "Motors"() -> ("Motor"=w1411:cluster{"Port":T4, "Port":T4})
                n313 = xnode "Motors"() -> ("Motor"=w1408:T4)
                n314 = xnode "Stop Motors"("Motors"=w1411) -> ()  [unwired: 1 in, 1 out]
                n315 = xnode "Move a Fixed Distance"("Speed 1"=i8 40, "Distance 1"=w1405, "Motors"=w1408) -> ("NXT/EV3"=w1407:T7)  [unwired: 1 in]
                n316 = xnode "Motor Status"("Motors"=w1408, "NXT/EV3"=w1407) -> ("Position 1"=w1406:i32)  [unwired: 2 out]
                n317 = Greater Or Equal?(x=w1406, y=w1405) -> (x >= y?=w1404:bool)
                n318 = Select(t=T3."end", s=w1404, f=T3."return") -> (s? t:f=w1401:T3)
              }
              frame "end" {
                n319 = xnode "Motors"() -> ("Motor"=w1438:cluster{"Port":T4, "Port":T4, "Port":T4})
                n320 = xnode "Stop Motors"("Motors"=w1438) -> ()  [unwired: 1 in, 1 out]
              }
            }
            n321 = Equal?(x=w1252, y=T2."Reference_pos") -> (x = y?=w1251:bool)
          }
        }
        frame True {
          n322 = Replace Array Subset(array=w1449, new element=1 ("new element/subarray"), index=0) -> (w1448:i32[])
          n323 = while {
            shift-right: [w1459] -> _
            shift-left: T6."forward" -> [w1458]
            tunnel: [w1454] -> w1452
            stop <- w1456 stop-if-true
            n324 = case shown="\"forward\", Default" w1458 {
              tunnel: [w1460 w1503 T6."up" w1545 w1577 _] -> w1459
              tunnel: [w1469 w1496 w1528 w1539 w1585 w1612] -> w1457
              tunnel: [w1469 w1496 w1528 w1539 w1585 w1612] -> w1454
              frame "forward", Default {
                w1465 = -3000 ("Distance 1")
                w1469 = T2."move4"
                n325 = xnode "Motors"() -> ("Motor"=w1464:T4)
                n326 = xnode "Motors"() -> ("Motor"=w1470:cluster{"Port":T4, "Port":T4})
                n327 = xnode "Stop Motors"("Motors"=w1470) -> ()  [unwired: 1 in, 1 out]
                n328 = xnode "Move a Fixed Distance"("Speed 1"=i8 -40, "Distance 1"=w1465, "Motors"=w1464) -> ("NXT/EV3"=w1466:T7)  [unwired: 1 in]
                n329 = xnode "Motor Status"("Motors"=w1464, "NXT/EV3"=w1466) -> ("Position 1"=w1467:i32)  [unwired: 2 out]
                n330 = Less Or Equal?(x=w1467, y=w1465) -> (x <= y?=w1463:bool)
                n331 = Select(t=T6."mark", s=w1463, f=T6."forward") -> (s? t:f=w1460:T6)
              }
              frame "mark" {
                w1496 = T2."move4"
                n332 = xnode "Motors"() -> ("Motor"=w1505:cluster{"Port":T4, "Port":T4})
                n333 = xnode "Motors"() -> ("Motor"=w1500:T4)
                n334 = xnode "Move Motors"("Power/Speed 1"=i8 -10, "Motors"=w1500) -> ()  [unwired: 1 in, 1 out]
                n335 = xnode "Stop Motors"("Motors"=w1505) -> ()  [unwired: 1 in, 1 out]
                n336 = xnode "Motor Status"("Motors"=w1500) -> ("Position 1"=w1499:i32)  [unwired: 1 in, 2 out]
                n337 = Less Or Equal?(x=w1499, y=0) -> (x <= y?=w1497:bool)
                n338 = Select(t=T6."pause", s=w1497, f=T6."mark") -> (s? t:f=w1503:T6)
              }
              frame "pause" {
                w1528 = T2."move4"
                n339 = xnode "Motors"() -> ("Motor"=w1531:cluster{"Port":T4, "Port":T4, "Port":T4})
                n340 = Wait (ms)(milliseconds to wait=u32 500 ("millisecond timer value")) -> ()  [unwired: 1 out]
                n341 = xnode "Stop Motors"("Motors"=w1531) -> ()  [unwired: 1 in, 1 out]
              }
              frame "up" {
                w1539 = T2."move4"
                n342 = xnode "Motors"() -> ("Motor"=w1547:cluster{"Port":T4, "Port":T4})
                n343 = xnode "Motors"() -> ("Motor"=w1538:T4)
                n344 = xnode "Motors"() -> ("Motor"=w1541:T4)
                n345 = xnode "Reset Encoders"("Motors"=w1538) -> ()  [unwired: 1 in, 1 out]
                n346 = xnode "Move Motors"("Power/Speed 1"=i8 10, "Motors"=w1541) -> ()  [unwired: 1 in, 1 out]
                n347 = xnode "Stop Motors"("Motors"=w1547) -> ()  [unwired: 1 in, 1 out]
                n348 = xnode "Motor Status"("Motors"=w1541) -> ("Position 1"=w1542:i32)  [unwired: 1 in, 2 out]
                n349 = Greater Or Equal?(x=w1542, y=100) -> (x >= y?=w1546:bool)
                n350 = Select(t=T6."return", s=w1546, f=T6."up") -> (s? t:f=w1545:T6)
              }
              frame "return" {
                w1580 = 2500 ("Distance 1")
                w1585 = T2."move4"
                n351 = xnode "Motors"() -> ("Motor"=w1586:cluster{"Port":T4, "Port":T4})
                n352 = xnode "Motors"() -> ("Motor"=w1583:T4)
                n353 = xnode "Stop Motors"("Motors"=w1586) -> ()  [unwired: 1 in, 1 out]
                n354 = xnode "Move a Fixed Distance"("Speed 1"=i8 40, "Distance 1"=w1580, "Motors"=w1583) -> ("NXT/EV3"=w1582:T7)  [unwired: 1 in]
                n355 = xnode "Motor Status"("Motors"=w1583, "NXT/EV3"=w1582) -> ("Position 1"=w1581:i32)  [unwired: 2 out]
                n356 = Greater Or Equal?(x=w1581, y=w1580) -> (x >= y?=w1576:bool)
                n357 = Select(t=T6."end", s=w1576, f=T6."return") -> (s? t:f=w1577:T6)
              }
              frame "end" {
                w1612 = T2."Reference_pos"
                n358 = xnode "Motors"() -> ("Motor"=w1613:cluster{"Port":T4, "Port":T4, "Port":T4})
                n359 = xnode "Stop Motors"("Motors"=w1613) -> ()  [unwired: 1 in, 1 out]
              }
            }
            n360 = Equal?(x=w1457, y=T2."Reference_pos") -> (x = y?=w1456:bool)
          }
        }
      }
    }
  }
  "Array out" <- w9
  "Array 4" <- w7
  "Array 5" <- w6
  "Enum out" <- w3
  "Enum 3" <- w2
